vi "ziExample-LabOne-GettingStarted.vi"   [LabVIEW 2009]
doc: "Control a Zurich instrument device via the LabOne Labview API. \nGetting started guide for Zurich Instruments Series: \n- quick overview for experts \n- easy introduction for LabVIEW beginners\n\n© Zurich Instruments AG, www.zhinst.com"
panel:
  # "Getting Started"
  # "SEE DIAGRAM\nFOR VI TREE.\n(CTRL+E)"
  # "(c) 2010-2014 Zurich Instruments.  ALL RIGHTS RESERVED."
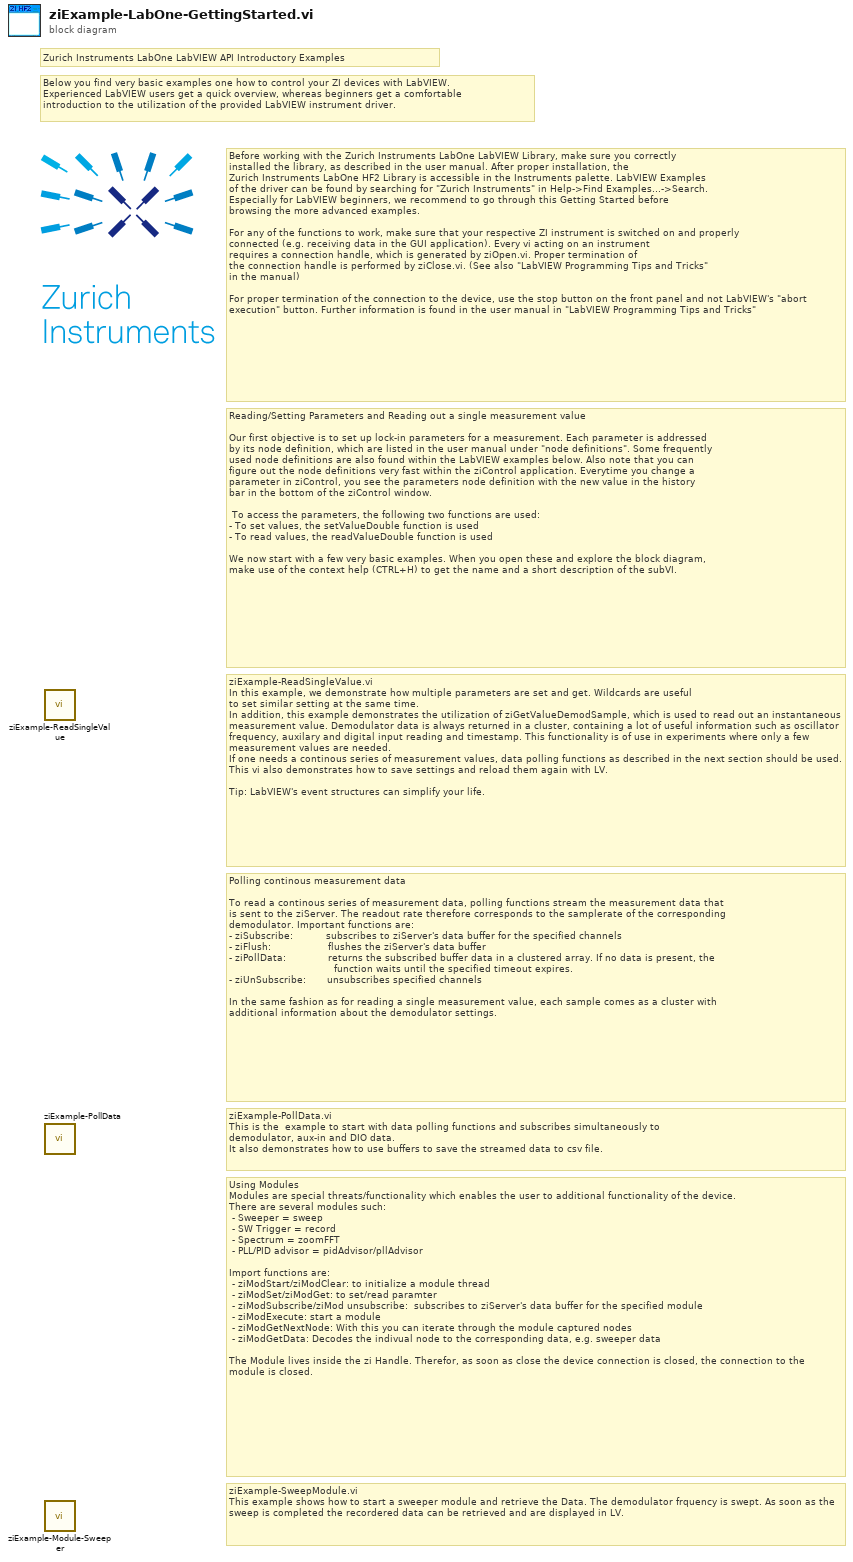
[diagram p0: block diagram]
diagram:
  # "ziExample-SweepModule.vi\nThis example shows how to start a sweeper module and retrieve the Data. The demodulator frquency is swept. As soon as the sweep is completed the recordered data can be retrieved and are displayed in LV."
  # "Using Modules\nModules are special threats/functionality which enables the user to additional functionality of the device.\nThere are several modules such:\n - Sweeper = sweep\n - SW Trigger = record\n - Spectrum = zoomFFT \n - PLL/PID advisor = pidAdvisor/pllAdvisor\n\nImport functions are:\n - ziModStart/ziModClear: to initialize a module thread\n - ziModSet/ziModGet: to set/read paramter\n - ziModSubscribe/ziMod unsubscribe:  subscribes to ziServer's data buffer for the specified module\n - ziModExecute: start a module\n - ziModGetNextNode: With this you can iterate through the module captured nodes\n - ziModGetData: Decodes the indivual node to the corresponding data, e.g. sweeper data\n\nThe Module lives inside the zi Handle. Therefor, as soon as close the device connection is closed, the connection to the module is closed."
  # "Zurich Instruments LabOne LabVIEW API Introductory Examples"
  # "Below you find very basic examples one how to control your ZI devices with LabVIEW. \nExperienced LabVIEW users get a quick overview, whereas beginners get a comfortable \nintroduction to the utilization of the provided LabVIEW instrument driver."
  # "Reading/Setting Parameters and Reading out a single measurement value\n\nOur first objective is to set up lock-in parameters for a measurement. Each parameter is addressed\nby its node definition, which are listed in the user manual under \"node definitions\". Some frequently\nused node definitions are also found within the LabVIEW examples below. Also note that you can \nfigure out the node definitions very fast within the ziControl application. Everytime you change a \nparameter in ziControl, you see the parameters node definition with the new value in the history\nbar in the bottom of the ziControl window.\n\n To access the parameters, the following two functions are used:\n- To set values, the setValueDouble function is used\n- To read values, the readValueDouble function is used\n\nWe now start with a few very basic examples. When you open these and explore the block diagram, \nmake use of the context help (CTRL+H) to get the name and a short description of the subVI."
  # "Before working with the Zurich Instruments LabOne LabVIEW Library, make sure you correctly \ninstalled the library, as described in the user manual. After proper installation, the\nZurich Instruments LabOne HF2 Library is accessible in the Instruments palette. LabVIEW Examples \nof the driver can be found by searching for \"Zurich Instruments\" in Help->Find Examples...->Search. \nEspecially for LabVIEW beginners, we recommend to go through this Getting Started before \nbrowsing the more advanced examples.\n\nFor any of the functions to work, make sure that your respective ZI instrument is switched on and properly \nconnected (e.g. receiving data in the GUI application). Every vi acting on an instrument\nrequires a connection handle, which is generated by ziOpen.vi. Proper termination of\nthe connection handle is performed by ziClose.vi. (See also \"LabVIEW Programming Tips and Tricks\"\nin the manual)\n\nFor proper termination of the connection to the device, use the stop button on the front panel and not LabVIEW's \"abort execution\" button. Further information is found in the user manual in \"LabVIEW Programming Tips and Tricks\""
  # "ziExample-PollData.vi\nThis is the  example to start with data polling functions and subscribes simultaneously to \ndemodulator, aux-in and DIO data. \nIt also demonstrates how to use buffers to save the streamed data to csv file."
  # "Polling continous measurement data\n\nTo read a continous series of measurement data, polling functions stream the measurement data that \nis sent to the ziServer. The readout rate therefore corresponds to the samplerate of the corresponding \ndemodulator. Important functions are:\n- ziSubscribe:           subscribes to ziServer's data buffer for the specified channels\n- ziFlush:                   flushes the ziServer's data buffer\n- ziPollData:              returns the subscribed buffer data in a clustered array. If no data is present, the \n                                   function waits until the specified timeout expires.\n- ziUnSubscribe:       unsubscribes specified channels\n\nIn the same fashion as for reading a single measurement value, each sample comes as a cluster with \nadditional information about the demodulator settings."
  # "ziExample-ReadSingleValue.vi\nIn this example, we demonstrate how multiple parameters are set and get. Wildcards are useful \nto set similar setting at the same time. \nIn addition, this example demonstrates the utilization of ziGetValueDemodSample, which is used to read out an instantaneous measurement value. Demodulator data is always returned in a cluster, containing a lot of useful information such as oscillator frequency, auxilary and digital input reading and timestamp. This functionality is of use in experiments where only a few measurement values are needed. \nIf one needs a continous series of measurement values, data polling functions as described in the next section should be used.\nThis vi also demonstrates how to save settings and reload them again with LV.\n\nTip: LabVIEW's event structures can simplify your life."
  n1 = call <instrlib>:"ziExample-ReadSingleValue.vi"() -> ()  [unwired: 23 in, 5 out]
  n2 = call <instrlib>:"ziExample-PollData.vi"() -> ()  [unwired: 19 in, 9 out]
  n3 = call <instrlib>:"ziExample-Module-Sweeper.vi"() -> ()  [unwired: 1 in]
